vi "Update Row Headers.vi"(0 "Test Table":refnum<vi>) -> ()   [LabVIEW 2018]
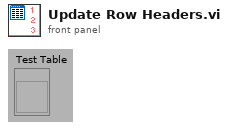
[diagram p1: front panel]
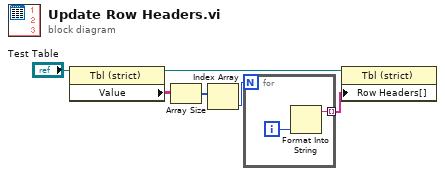
[diagram p0: block diagram]
diagram:
  n1 = property class="Tbl (strict)"(reference="Test Table") -> (reference out=w4:refnum<vi>, "Value"=w3:string[][])  [unwired: 1 in, 1 out]
  n2 = Array Size(array=w3) -> (size(s)=w2:i32[])
  n3 = Index Array(array=w2) -> (element=w1:i32)  [unwired: 1 in]
  n4 = for {
    N: w1 -> [_]
    tunnel: [w7] -> w5 mode=indexing
    i -> [w8]
    n5 = Format Into String(w8) -> (resulting string=w7:string)  [unwired: 3 in, 1 out]
  }
  n6 = property class="Tbl (strict)"(reference=w4, "Row Headers[]"=w5) -> ()  [unwired: 1 in, 2 out]
